vi "SQL edit expt device variable.vi"(6 "Variable Name":string, 9 "Device ID":string, 10 "Corresponding values":string[](array[string]), 11 "Columns":string[](array[string])) -> (0 "error out":errorcluster)   [LabVIEW 2013]
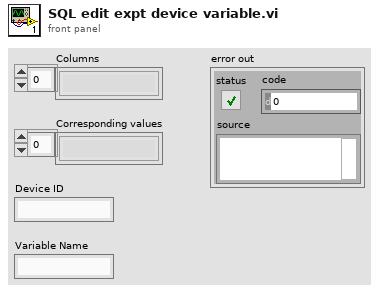
[diagram p1: front panel]
types:
  T1 = typedef "mysql_authentication.ctl" = cluster{"User":string, "Password":string, "Database":string}
  T2 = cluster{"Port":u16, "IP Address":string, "Authentication":T1}
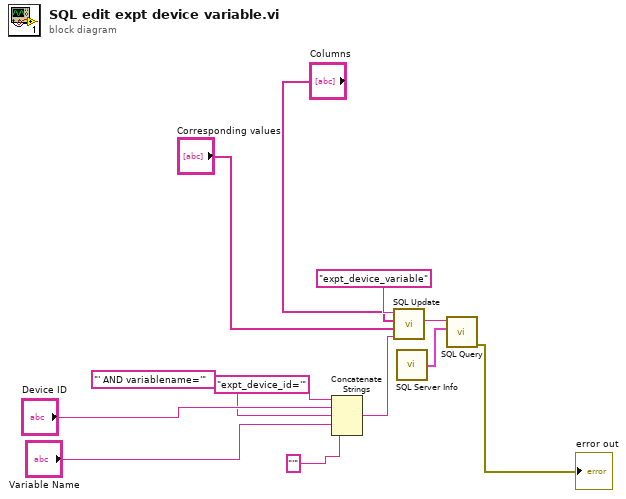
[diagram p0: block diagram]
diagram:
  n1 = Concatenate Strings("expt_device_id='" ("string"), "Device ID", "' AND variablename='" ("Query String"), "Variable Name", "'") -> (w4:string)
  n2 = call "SQL Update.vi"("Where clause"=w4, "Values"="Corresponding values", "Column Names"="Columns", "Table"="expt_device_variable") -> ("Query String"=w8:string)  [unwired: 7 in]
  n3 = call "SQL Server Info.vi"() -> ("SQL Server Info"=w2:T2)
  n4 = call "SQL Query.vi"("SQL Server Info"=w2, "Query"=w8) -> ("error out"=→"error out":errorcluster)  [unwired: 8 in, 1 out]
